vi "Voltage and Current Ring Chooser.vi"(8 "error in (no error)":errorcluster, 11 "Universal Power Meter in":refnum<class "Universal Power Meter.lvclass">) -> (0 "error out":errorcluster, 1 "Current Strings And Values []":T1, 2 "Voltage Strings And Values []":T1, 3 "Universal Power Meter out":refnum<class "Universal Power Meter.lvclass">, 4 "Wiring Strings And Values []":T1)   [LabVIEW 2013, in "Universal Power Meter.lvlib" / "Universal Power Meter.lvclass"]
uses:
  Universal Power Meter.lvclass
  <vilib>/Utility/miscctls.llb/LVStringsAndValuesArrayTypeDef_U16.ctl
  Generic Instrument/Generic Instrument.lvclass
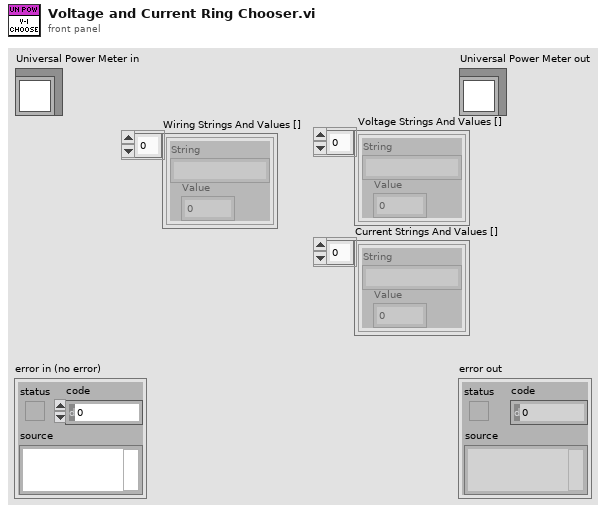
[diagram p1: front panel]
types:
  T1 = typedef "LVStringsAndValuesArrayTypeDef_U16.ctl" = cluster{"String":string, "Value":u16}[]
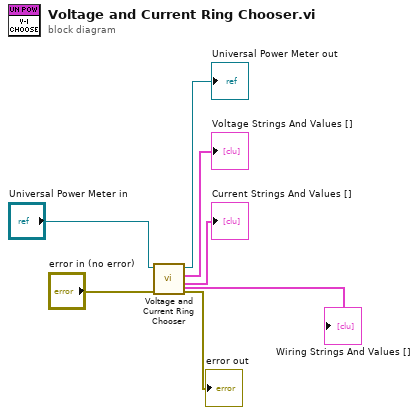
[diagram p0: block diagram]
diagram:
  n1 = call-parent "Voltage and Current Ring Chooser.vi"("error in (no error)"="error in (no error)", "Generic Instrument in"="Universal Power Meter in") -> ("error out"=→"error out":errorcluster, "Current Strings And Values []"=→"Current Strings And Values []":T1, "Voltage Strings And Values []"=→"Voltage Strings And Values []":T1, "Generic Instrument out"=→"Universal Power Meter out":refnum<class "Universal Power Meter.lvclass">, "Wiring Strings And Values []"=→"Wiring Strings And Values []":T1)  [unwired: 5 in]
